vi "write_ini.vi"(8 "error in (no error)":errorcluster caption="错误输入（无错误）", 9 "section name":string, 10 "file ref in":T1, 11 "MotorSystem 输入":refnum<class "MotorSystem.lvclass">) -> (0 "error out":errorcluster caption="错误输出", 2 "file ref out":T1, 3 "MotorSystem 输出":refnum<class "MotorSystem.lvclass">)   [LabVIEW 2016, in "MotionControl_UFO_3DOF.lvlib" / "MotorSystem.lvclass"]
uses:
  <userlib>/MotionControl_UFO_3DOF/MotorSystem/MotorSystem.lvclass
  <vilib>/Utility/config.llb/Config Data RefNum.ctl
  <userlib>/MotionControl_UFO_3DOF/MotorSystem/MotorSystem.lvclass/MotorSystem.ctl
  <vilib>/Utility/config.llb/Write Key (String).vi
  <vilib>/Utility/config.llb/Write Key (U32).vi
  <vilib>/Utility/config.llb/Write Key (I32).vi
  <vilib>/Utility/config.llb/Write Key (Boolean).vi
  <vilib>/Utility/error.llb/Error Cluster From Error Code.vi
  <vilib>/ErrorRing/Error Ring.xnode
  <userlib>/MotionControl_UFO_3DOF/OneMotion/OneMotion.lvclass
  <vilib>/Utility/config.llb/NI_LVConfig.lvlib
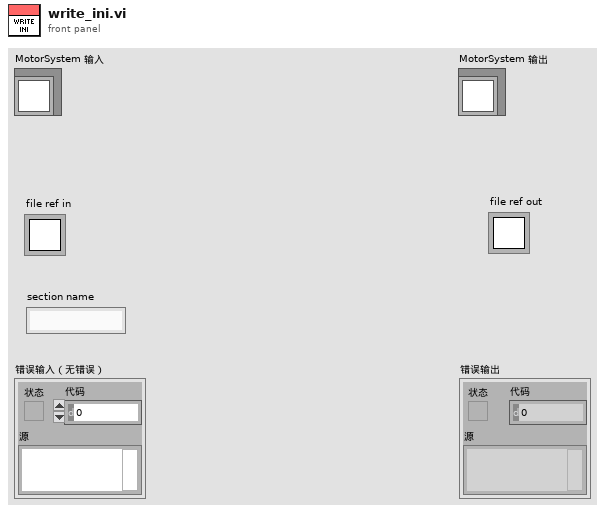
[diagram p1: front panel]
types:
  T1 = typedef "NI_LVConfig.lvlib/Config Data RefNum.ctl" = refnum<k1>
  T2 = typedef "MotionControl_UFO_3DOF.lvlib/MotorSystem.lvclass/MotionCluster.ctl" = cluster{"OneMotion.lvclass":refnum<class "OneMotion.lvclass">, "connected?":bool, "default enabled?":bool, "enabled?":bool}
  T3 = typedef "MotionControl_UFO_3DOF.lvlib/StepMotor.lvclass/DEV_INFO.ctl" = cluster{"设备类型(0x01 = RS232CAN;0x02 = WIFI2RS232CAN;0x04 = USBCAN)":u32, "设备编号":u32, "系统为RS232CAN网关设备分配的COM口编号，这个成员变量只对\nRS232网关设备有用":u32, "RS232CAN网关设备与PC通讯的串口波特率，这个成员变量只对\nRS232网关设备有用":u32, "保存网关设备的名称":string}
  T4 = cluster{"complete dimension names":string[], "dimension names cluster ":cluster{"name 1":string, "name 2":string, "name 3":string}}
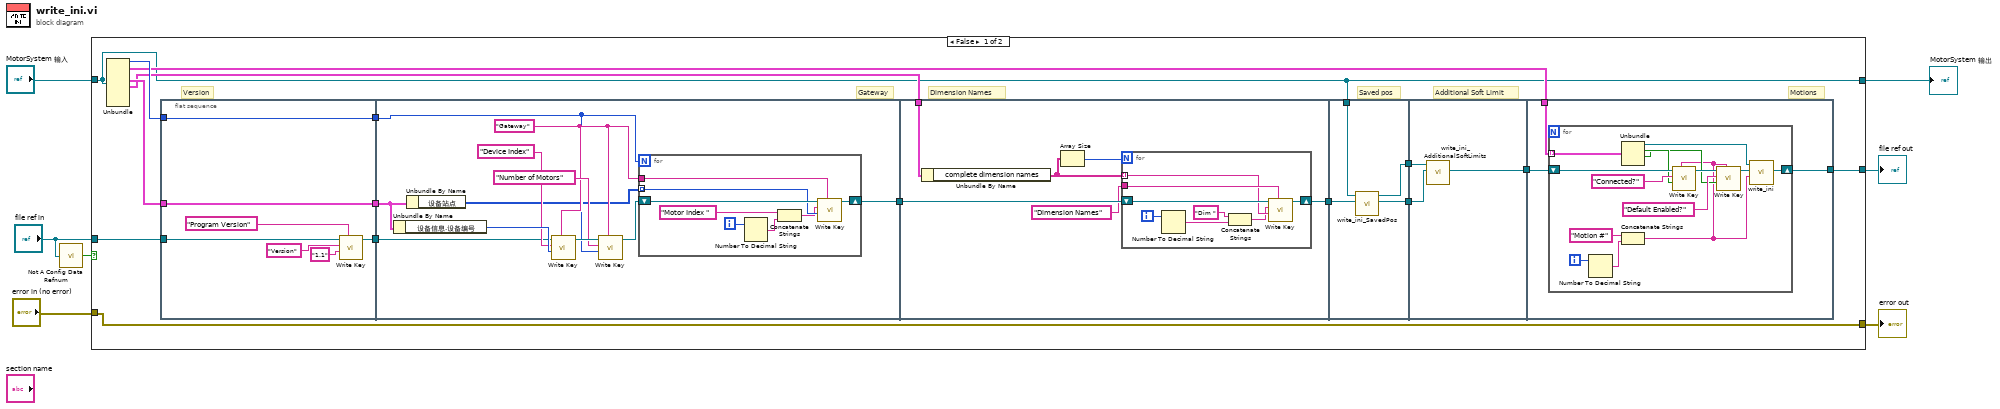
[diagram p0: block diagram]
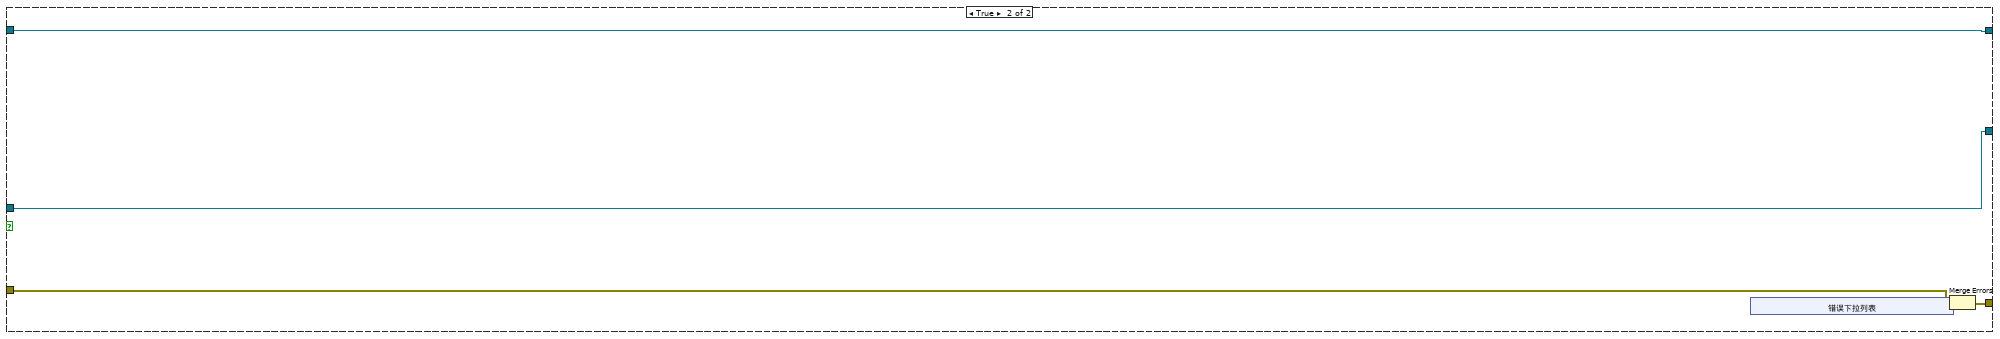
[diagram p2: hidden frame]
diagram:
  n1 = call <vilib>:"Not A Config Data Refnum.vi"("refnum"="file ref in") -> ("not a config data refnum"=w1:bool)
  n2 = case shown="False" w1 {
    tunnel: [w23 w88] -> w7
    tunnel: [w11 w91] -> w5
    tunnel: "MotorSystem 输入" -> [w11 w91]
    tunnel: "file ref in" -> [w22 w92]
    tunnel: [w17 w92] -> w3
    tunnel: "error in (no error)" -> [w23 w89]
    frame False {
      # "Additional Soft Limit"
      # "Saved pos"
      # "Dimension Names"
      # "Version"
      # "Motions"
      # "Gateway"
      n3 = Unbundle(w11) -> (w21:i32, w12:T2[], w20:cluster{"CAN 波特率":u32, "设备信息":T3, "设备站点":u32[]}, w18:T4)  [unwired: 4 out]
      n4 = flat-sequence {
        tunnel: w20 -> [w29]
        tunnel: w21 -> [w30]
        tunnel: w22 -> [w28]
        tunnel: [w27] -> w16
        tunnel: [w30] -> w15
        tunnel: [w29] -> w14
        tunnel: [w31] -> w19
        tunnel: w16 -> [w39]
        tunnel: w15 -> [w34]
        tunnel: w14 -> [w33]
        tunnel: w19 -> [w53]
        tunnel: w18 -> [w54]
        tunnel: [w52] -> w13
        tunnel: w13 -> [w66]
        tunnel: [w65] -> w10
        tunnel: w11 -> [w67]
        tunnel: [w64] -> w8
        tunnel: w10 -> [w69]
        tunnel: [w68] -> w9
        tunnel: w8 -> [w70]
        tunnel: [w72] -> w17
        tunnel: w9 -> [w73]
        tunnel: w12 -> [w71]
        frame #0 {
          n5 = call-poly <vilib>:"Write Key.vi"("section"="Program Version", "value"="1.1", "key"="Version", "refnum"=w28) -> ("refnum out"=w27:T1)  [unwired: 5 in, 2 out]
        }
        frame #1 {
          w36 = "Gateway"
          n6 = Unbundle By Name(w33) -> ("设备信息.设备编号"=w41:u32)
          n7 = Unbundle By Name(w33) -> ("设备站点"=w32:u32[])
          n8 = call-poly <vilib>:"Write Key.vi"("section"=w36, "value"=w41, "key"="Device Index", "refnum"=w39) -> ("refnum out"=w38:T1)  [unwired: 5 in, 2 out]
          n9 = call-poly <vilib>:"Write Key.vi"("section"=w36, "value"=w34, "key"="Number of Motors", "refnum"=w38) -> ("refnum out"=w35:T1)  [unwired: 5 in, 2 out]
          n10 = for {
            N: w34 -> [_]
            tunnel: w36 -> [w49]
            shift-right: [w47] -> w31
            shift-left: w35 -> [w48]
            tunnel: w32 -> [w46] mode=indexing
            i -> [w45]
            n11 = Number To Decimal String(number=w45) -> (decimal integer string=w43:string)  [unwired: 1 in]
            n12 = Concatenate Strings("Motor Index ", w43) -> (w42:string)
            n13 = call-poly <vilib>:"Write Key.vi"("section"=w49, "value"=w46, "key"=w42, "refnum"=w48) -> ("refnum out"=w47:T1)  [unwired: 5 in, 2 out]
          }
        }
        frame #2 {
          n14 = Unbundle By Name(w54) -> ("complete dimension names"=w50:string[])
          n15 = Array Size(array=w50) -> (size(s)=w55:i32)
          n16 = for {
            N: w55 -> [_]
            tunnel: w50 -> [w60] mode=indexing
            shift-right: [w62] -> w52
            shift-left: w53 -> [w63]
            tunnel: "Dimension Names" -> [w61]
            i -> [w59]
            n17 = Number To Decimal String(number=w59) -> (decimal integer string=w58:string)  [unwired: 1 in]
            n18 = Concatenate Strings("Dim ", w58) -> (w56:string)
            n19 = call-poly <vilib>:"Write Key.vi"("section"=w61, "value"=w60, "key"=w56, "refnum"=w63) -> ("refnum out"=w62:T1)  [unwired: 5 in, 2 out]
          }
        }
        frame #3 {
          n20 = call <userlib>:"write_ini_SavedPos.vi"("file ref in"=w66, "MotorSystem 输入"=w67) -> ("file ref out"=w65:T1, "MotorSystem 输出"=w64:refnum<class "MotorSystem.lvclass">)  [unwired: 7 in, 1 out]
        }
        frame #4 {
          n21 = call <userlib>:"write_ini_AdditionalSoftLimits.vi"("file ref in"=w69, "MotorSystem 输入"=w70) -> ("file ref out"=w68:T1)  [unwired: 7 in, 2 out]
        }
        frame #5 {
          n22 = for {
            tunnel: w71 -> [w87] mode=indexing
            shift-right: [w85] -> w72
            shift-left: w73 -> [w80]
            i -> [w84]
            n23 = Number To Decimal String(number=w84) -> (decimal integer string=w83:string)  [unwired: 1 in]
            n24 = Unbundle(w87) -> ("OneMotion.lvclass"=w86:refnum<class "OneMotion.lvclass">, "connected?"=w79:bool, "default enabled?"=w76:bool)  [unwired: 1 out]
            n25 = Concatenate Strings("Motion #", w83) -> (w75:string)
            n26 = call-poly <vilib>:"Write Key.vi"("section"=w75, "value"=w79, "key"="Connected?", "refnum"=w80) -> ("refnum out"=w78:T1)  [unwired: 5 in, 2 out]
            n27 = call-poly <vilib>:"Write Key.vi"("section"=w75, "value"=w76, "key"="Default Enabled?", "refnum"=w78) -> ("refnum out"=w74:T1)  [unwired: 5 in, 2 out]
            n28 = call-dynamic "write_ini.vi"("section name"=w75, "file ref in"=w74, "OneMotion 输入"=w86) -> ("file ref out"=w85:T1)  [unwired: 6 in, 2 out]
          }
        }
      }
    }
    frame True {
      n29 = xnode "错误下拉列表"() -> ("error out"=w90:errorcluster)
      n30 = Merge Errors(w89, w90) -> (w88:errorcluster)
    }
  }
  "error out" <- w7
  "MotorSystem 输出" <- w5
  "file ref out" <- w3
